vi "Microscope Base Control.vi"() -> ()   [LabVIEW 2020]
uses:
  <vilib>/Utility/miscctls.llb/LVPointTypeDef.ctl
panel:
  in  "Setup Base":bool
  in  "Lock Base":bool
  in  "Lamp Power (%)":u16
  in  "Lamp On/Off":bool
  in  "Output Port":T1(radio)
  in  "Lamp":u8(ring) items=["Lamp 01", "Lamp 02", "Lamp 03"]
  in  "Turrent Filter":T2(radio)
  in  "Lock Focus Knob":bool
  in  "Escape":bool
  in  "Step 8":bool
  in  "Step 7":bool
  in  "Step 6":bool
  in  "Step 5":bool
  in  "Step 4":bool
  in  "Step 3":bool
  in  "Step 2":bool
  in  "Step 1":bool
  in  "Far/Out":bool
  in  "Near/In":bool
  in  "Position (µm)":dbl format="%#.3g"
  in  "Step Size (µm)":dbl=0.1
  in  "Objective Lens":T2(radio)
  in  "Calling VI Ref":refnum<vi>
  in  "Quit":bool
  # "Preset Step Sizes"
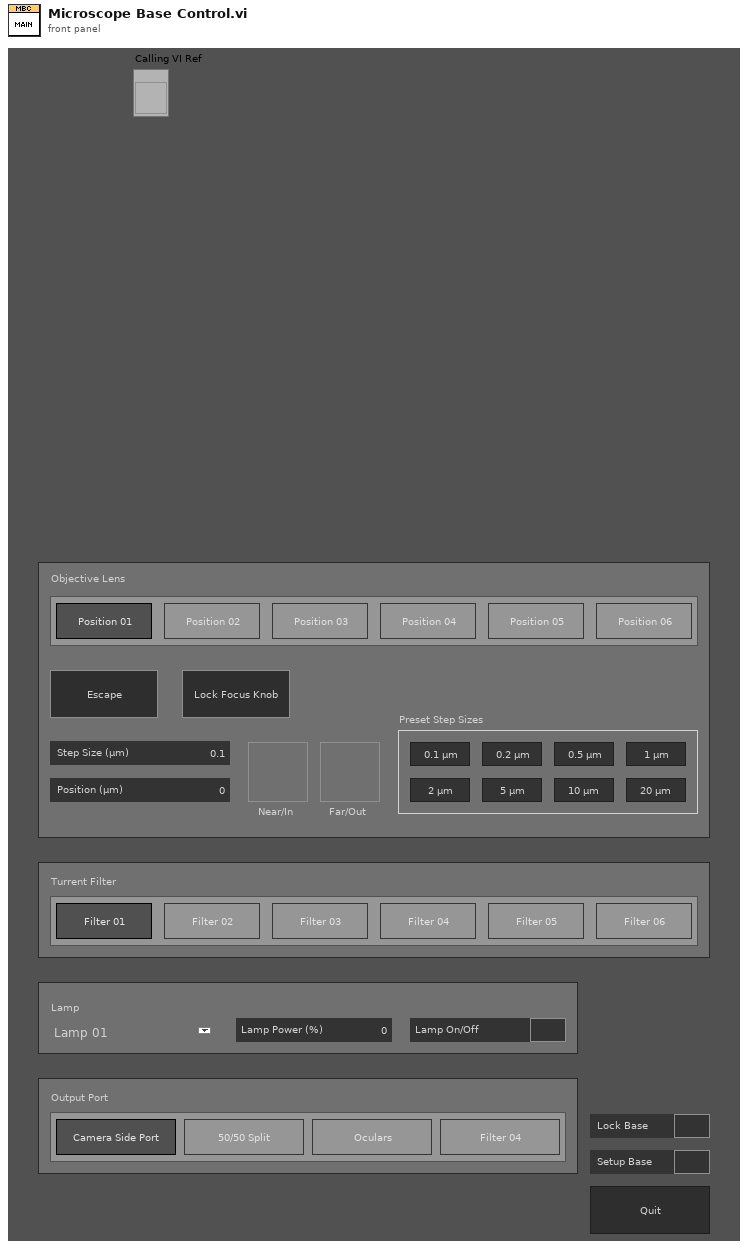
[diagram p1: front panel]
types:
  T1 = enum32{"Delay 01", "Delay 02", "Radio Selection 3", "Radio Selection 4"}
  T2 = enum32{"Delay 01", "Delay 02", "Radio Selection 3", "Radio Selection 4", "Radio Selection 5", "Radio Selection 6"}
  T3 = enum16{"Always On", "Always Off", "Off While Running"}
  T4 = typedef "LVPointTypeDef.ctl" = cluster{"Horizontal":i16, "Vertical":i16}
  T5 = typedef "LVRectTypeDef.ctl" = cluster{"Left":i16, "Top":i16, "Right":i16, "Bottom":i16}
  T6 = typedef "LVBoundsTypeDef.ctl" = cluster{"Width":u32, "Height":u32}
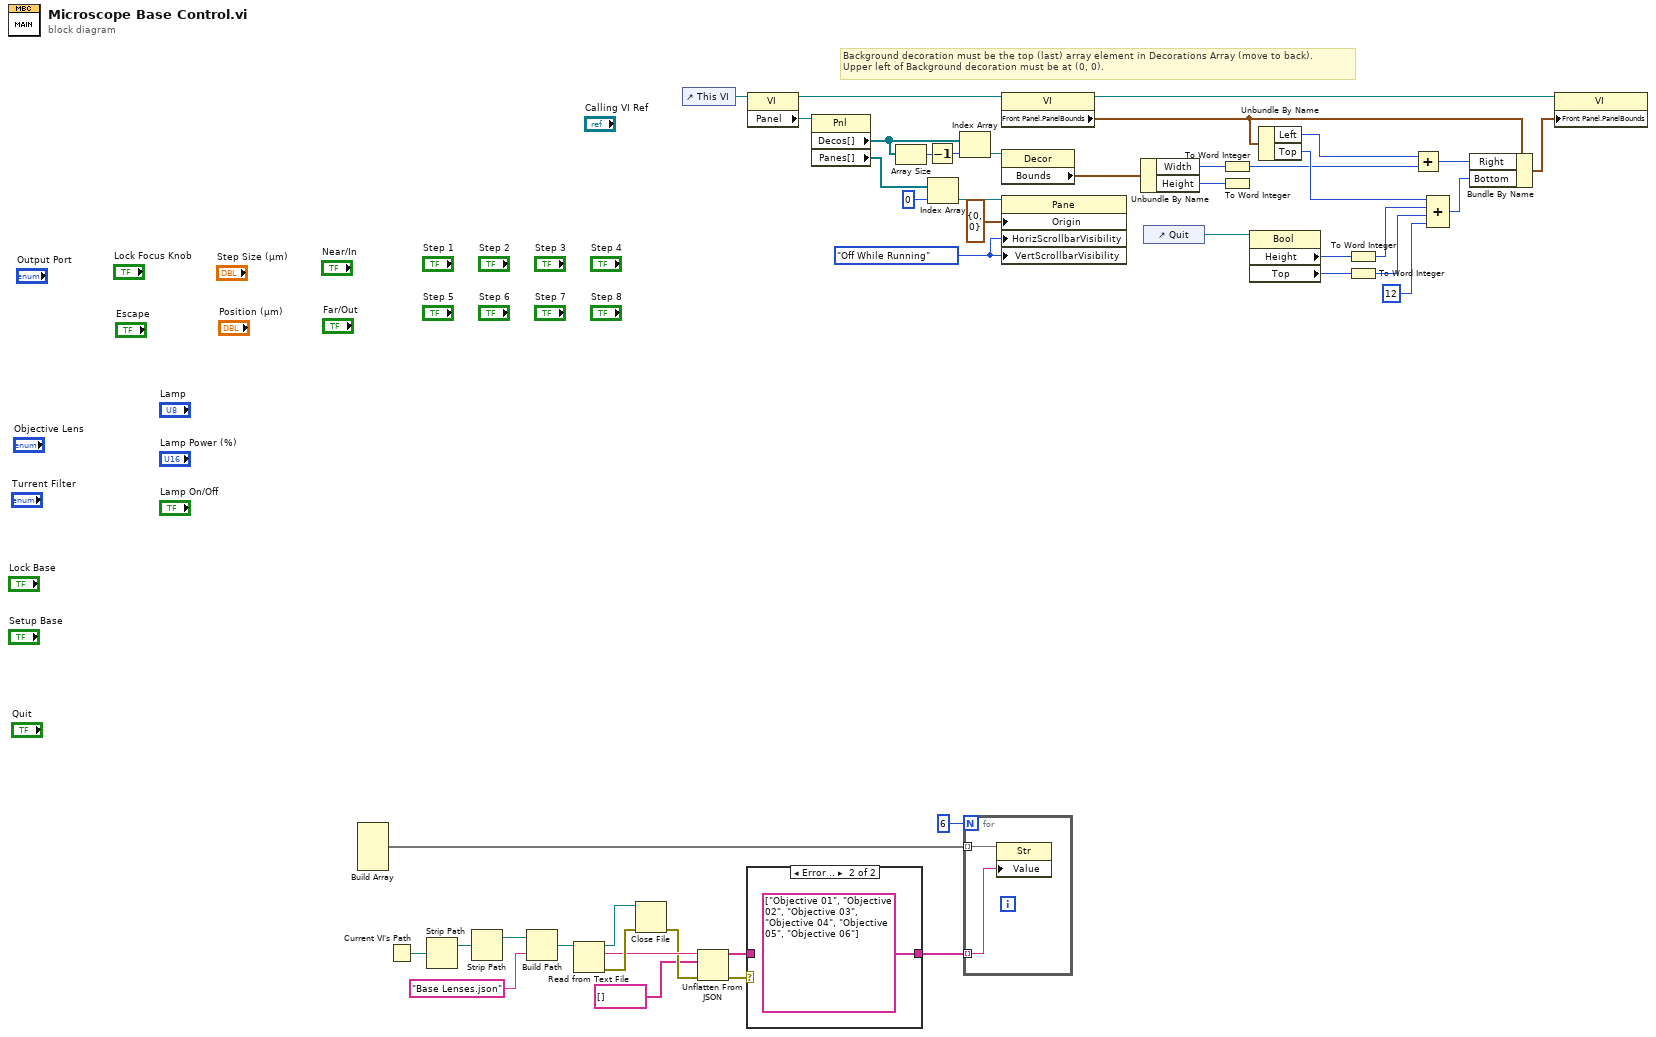
[diagram p0: block diagram]
diagram:
  w12 = T3."Off While Running" ("Vertical Scrollbar Visibility")
  # "Background decoration must be the top (last) array element in Decorations Array (move to back).\nUpper left of Background decoration must be at (0, 0)."
  n1 = Build Array() -> (w35:void[])  [unwired: 6 in]
  n2 = Current VI's Path() -> (path=w32:path)
  n3 = Strip Path(path=w32) -> (stripped path=w31:path)  [unwired: 1 out]
  n4 = Strip Path(path=w31) -> (stripped path=w44:path)  [unwired: 1 out]
  n5 = Build Path(base path=w44, name or relative path="Base Lenses.json") -> (appended path=w30:path)
  n6 = Read from Text File(file (use dialog)=w30) -> (refnum out=w42:refnum<file>, text=w40:string, error out=w41:errorcluster)  [unwired: 3 in, 1 out]
  n7 = Close File(refnum=w42, error in=w41) -> (error out=w39:errorcluster)  [unwired: 1 out]
  n8 = control-ref of="This VI"() -> (w4:refnum<vi>)
  n9 = Unflatten From JSON(JSON string=w40, type and defaults=string[] [], error in (no error)=w39) -> (value=w36:string[], error out=w37:errorcluster)  [unwired: 4 in]
  n10 = case shown="Error .." w37 {
    tunnel: w36 -> [w45 _]
    tunnel: [w45 string[] ["Objective 01", "Objective 02", "Objective 03", "Objective 04", "Objective 05", "Objective 06"]] -> w33
    frame No Error {
    }
    frame Error {
    }
  }
  n11 = property class="VI"(reference=w4) -> (reference out=w13:refnum<vi>, "Panel"=w5:refnum<vi>)  [unwired: 1 in, 1 out]
  n12 = property class="Pnl"(reference=w5) -> ("Decos[]"=w3:refnum<vi>[], "Panes[]"=w9:refnum<vi>[])  [unwired: 1 in, 2 out]
  n13 = Array Size(array=w3) -> (size(s)=w1:i32)
  n14 = Decrement(x=w1) -> (x-1=w2:i32)
  n15 = Index Array(array=w9, index=0) -> (element=w8:refnum<vi>)
  n16 = Index Array(array=w3, index=w2) -> (element=w11:refnum<vi>)
  n17 = for {
    N: 6 -> [_]
    tunnel: w35 -> [w48] mode=indexing
    tunnel: w33 -> [w47] mode=indexing
    n18 = property class="Str"(reference=w48, "Value"=w47) -> ()  [unwired: 1 in, 2 out]
  }
  n19 = property class="VI"(reference=w13) -> (reference out=w15:refnum<vi>, "Front Panel.PanelBounds"=w16:T5)  [unwired: 1 in, 1 out]
  n20 = property class="Decor"(reference=w11) -> ("Bounds"=w14:T6)  [unwired: 1 in, 2 out]
  n21 = property class="Pane"(reference=w8, "Origin"=T4 {"Horizontal"=0, "Vertical"=0}, "HorizScrollbarVisibility"=w12, "VertScrollbarVisibility"=w12) -> ()  [unwired: 1 in, 2 out]
  n22 = Unbundle By Name(w14) -> ("Width"=w19:u32, "Height"=w22:u32)
  n23 = control-ref of="Quit"() -> (w6:refnum<vi>)
  n24 = To Word Integer(number=w19) -> (16bit integer=w21:i16)
  n25 = To Word Integer(number=w22) -> ()  [unwired: 1 out]
  n26 = property class="Bool"(reference=w6) -> ("Height"=w24:u32, "Top"=w25:i32)  [unwired: 1 in, 2 out]
  n27 = Unbundle By Name(w16) -> ("Left"=w18:i16, "Top"=w29:i16)
  n28 = To Word Integer(number=w24) -> (16bit integer=w27:i16)
  n29 = To Word Integer(number=w25) -> (16bit integer=w28:i16)
  n30 = Add(x=w18, y=w21) -> (x+y=w20:i16)
  n31 = Compound Arithmetic op=ADD(w29, w27, w28, i16 12 ("y")) -> (w23:i16)
  n32 = Bundle By Name(cluster=w16, "Right"=w20, "Bottom"=w23) -> (w17:T5)
  n33 = property class="VI"(reference=w15, "Front Panel.PanelBounds"=w17) -> ()  [unwired: 1 in, 2 out]
